vi "Refresh DiffIO Listbox.vi"(4 "_DiffIOState":u8, 5 "AdaptMode":u32, 6 "Results":T1[](array[typedef]) {"Duty Cycle [%]" format="%#_3g"; "Frequency [Hz]" format="%#_3p"}, 7 "DigitalFilter":sgl[](array[numeric]) caption="Filters" format="%#.2p", 8 "Command":T2[](array[typedef]) {"Skip Fire Index" max=7; "Angles"."Duration [s]" format="%#_3p"; "Frequency [Hz]" format="%#_3p"}, 9 "Names":string[](array[string]), 11 "_DiffIO Channels":refnum<vi>) -> ()   [LabVIEW 2016]
uses:
  <vilib>/Powertrain Controls/Device Drivers/DCM/Diff IO/RT/Setup.ctl
  <vilib>/Powertrain Controls/Device Drivers/DCM/Diff IO/FPGA/Mode.ctl
  <vilib>/Powertrain Controls/Device Drivers/DCM/Diff IO/RT/Angle Control.ctl
  <vilib>/Powertrain Controls/Device Drivers/DCM/Diff IO/RT/Results.ctl
  <vilib>/Powertrain Controls/Device Drivers/DCM/Diff IO/RT/DCM - RT - Diff IO.lvlib
  <vilib>/Powertrain Controls/Device Drivers/DCM/Diff IO/FPGA/DCM - FPGA - Diff IO.lvlib
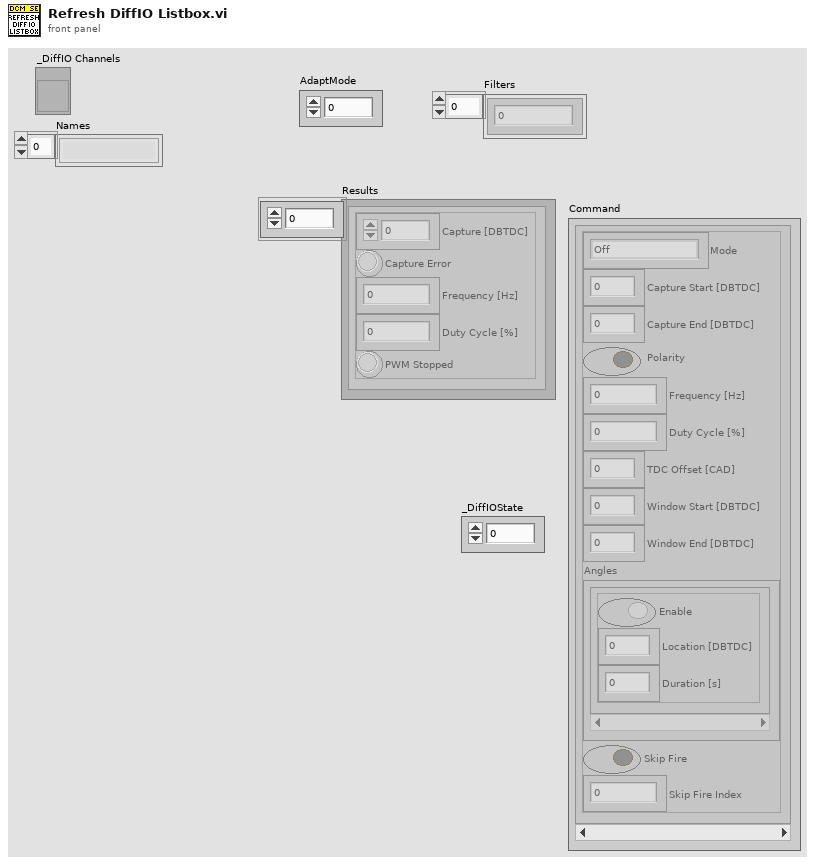
[diagram p1: front panel]
types:
  T1 = typedef "DCM - RT - Diff IO.lvlib/Results.ctl" = cluster{"Capture [DBTDC]":sgl, "Capture Error":bool, "Frequency [Hz]":sgl, "Duty Cycle [%]":sgl, "PWM Stopped":bool}
  T2 = typedef "DCM - RT - Diff IO.lvlib/Setup.ctl" = cluster{"Mode":T3, "Capture Start [DBTDC]":sgl, "Capture End [DBTDC]":sgl, "Polarity":bool, "Frequency [Hz]":sgl, "Duty Cycle [%]":sgl, "TDC Offset [CAD]":sgl, "Window Start [DBTDC]":sgl, "Window End [DBTDC]":sgl, "Angles":T4[], "Skip Fire":bool, "Skip Fire Index":u8}
  T3 = typedef "DCM - FPGA - Diff IO.lvlib/Mode.ctl" = enum8{"Off", "Input", "Pulse Width Modulation", "Engine Position Tracking", "Serial Out 1", "Serial Out 2"}
  T4 = typedef "DCM - RT - Diff IO.lvlib/Angle Control.ctl" = cluster{"Enable":bool, "Location [DBTDC]":sgl, "Duration [s]":sgl}
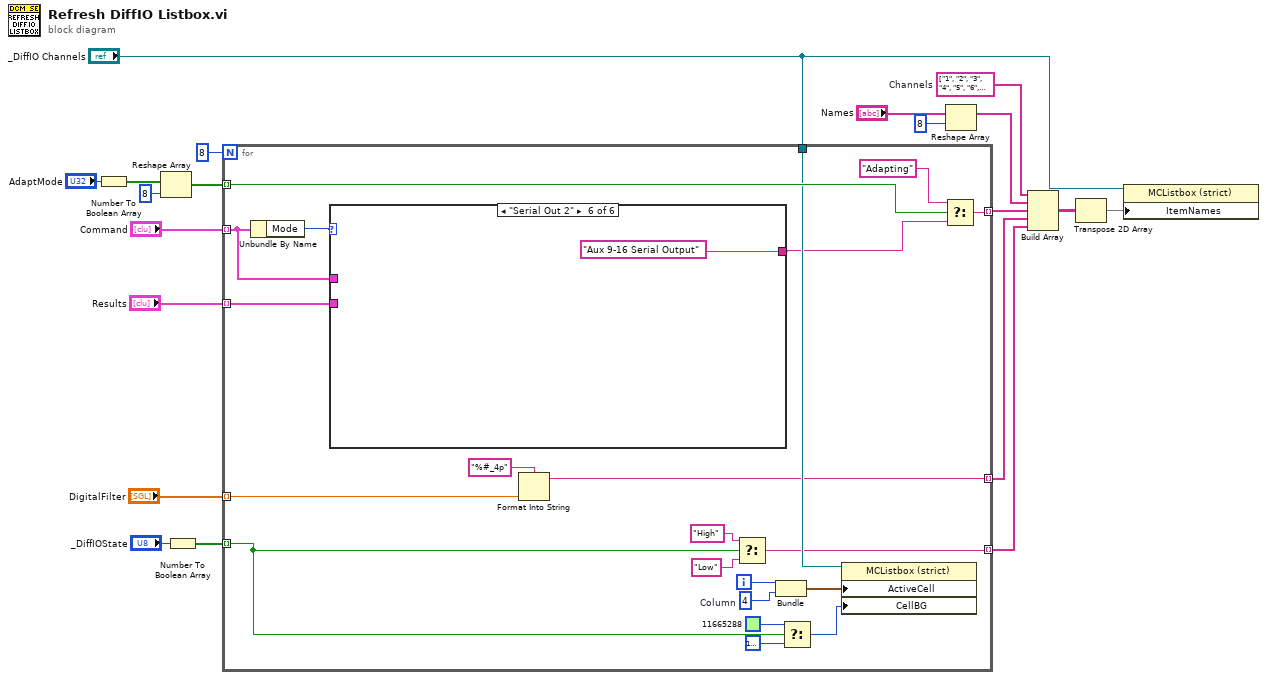
[diagram p0: block diagram]
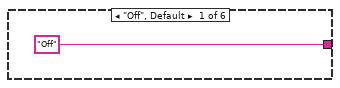
[diagram p2: hidden frame]
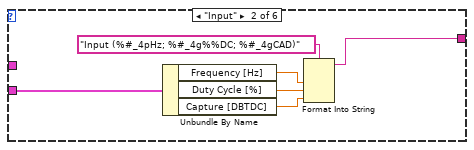
[diagram p3: hidden frame]
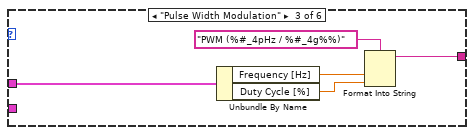
[diagram p4: hidden frame]
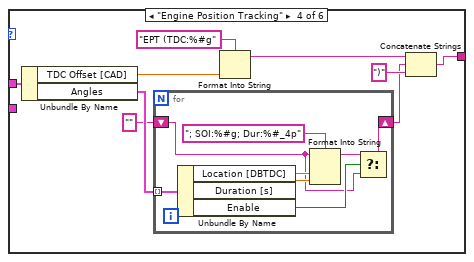
[diagram p5: hidden frame]
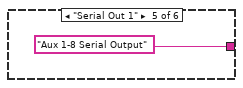
[diagram p6: hidden frame]
diagram:
  w18 = string[] ["1", "2", "3", "4", "5", "6", "7", "8"]  # Channels
  n1 = Number To Boolean Array(number="AdaptMode") -> (Boolean array=w11:bool[])
  n2 = Reshape Array(w11, 8 ("dimension size")) -> (w9:bool[])
  n3 = Number To Boolean Array(number="_DiffIOState") -> (Boolean array=w6:bool[])
  n4 = for {
    N: 8 -> [_]
    tunnel: "Command" -> [w26] mode=indexing
    tunnel: w9 -> [w40] mode=indexing
    tunnel: [w39] -> w8 mode=indexing
    tunnel: "Results" -> [w24] mode=indexing
    tunnel: w6 -> [w29] mode=indexing
    tunnel: [w28] -> w5 mode=indexing
    tunnel: "_DiffIO Channels" -> [w35]
    tunnel: "DigitalFilter" -> [w22] mode=indexing
    tunnel: [w23] -> w1 mode=indexing
    i -> [w37]
    w38 = 4  # Column
    n5 = Unbundle By Name(w26) -> ("Mode"=w27:T3)
    n6 = case shown="\"Serial Out 2\"" w27 {
      tunnel: w26 -> [_ _ w53 w61 _ _]
      tunnel: ["Off" w44 w49 w57 "Aux 1-8 Serial Output" ("format string") "Aux 9-16 Serial Output" ("format string")] -> w25
      tunnel: w24 -> [_ w43 _ _ _ _]
      frame "Off", Default {
      }
      frame "Input" {
        n7 = Unbundle By Name(w43) -> ("Frequency [Hz]"=w46:sgl, "Duty Cycle [%]"=w47:sgl, "Capture [DBTDC]"=w48:sgl)
        n8 = Format Into String(format string="Input (%#_4pHz; %#_4g%%DC; %#_4gCAD)", w46, w47, w48) -> (resulting string=w44:string)  [unwired: 2 in, 1 out]
      }
      frame "Pulse Width Modulation" {
        n9 = Unbundle By Name(w53) -> ("Frequency [Hz]"=w51:sgl, "Duty Cycle [%]"=w50:sgl)
        n10 = Format Into String(format string="PWM (%#_4pHz / %#_4g%%)", w51, w50) -> (resulting string=w49:string)  [unwired: 2 in, 1 out]
      }
      frame "Engine Position Tracking" {
        n11 = Unbundle By Name(w61) -> ("TDC Offset [CAD]"=w60:sgl, "Angles"=w59:T4[])
        n12 = for {
          tunnel: w59 -> [w68] mode=indexing
          shift-right: [w64] -> w55
          shift-left: "" -> [w63]
          n13 = Unbundle By Name(w68) -> ("Location [DBTDC]"=w69:sgl, "Duration [s]"=w67:sgl, "Enable"=w66:bool)
          n14 = Format Into String(format string="; SOI:%#g; Dur:%#_4p", initial string=w63, w69, w67) -> (resulting string=w65:string)  [unwired: 1 in, 1 out]
          n15 = Select(t=w65, s=w66, f=w63) -> (s? t:f=w64:string)
        }
        n16 = Format Into String(format string="EPT (TDC:%#g", w60) -> (resulting string=w58:string)  [unwired: 2 in, 1 out]
        n17 = Concatenate Strings(w58, w55, ")" ("string")) -> (w57:string)
      }
      frame "Serial Out 1" {
      }
      frame "Serial Out 2" {
      }
    }
    n18 = Format Into String(format string="%#_4p", w22) -> (resulting string=w23:string)  [unwired: 2 in, 1 out]
    n19 = Select(t="High" ("format string"), s=w29, f="Low" ("format string")) -> (s? t:f=w28:string)
    n20 = Bundle(w37, "Column"=w38) -> (w36:cluster{i32, "Column":i32})  [unwired: 1 in]
    n21 = Select(t=u32 11665288, s=w29, f=u32 16777226) -> (s? t:f=w32:u32)
    n22 = property on="Property Node" class="MCListbox (strict)"(reference=w35, "ActiveCell"=w36, "CellBG"=w32) -> ()  [unwired: 1 in, 2 out]
    n23 = Select(t="Adapting" ("format string"), s=w40, f=w25) -> (s? t:f=w39:string)
  }
  n24 = Reshape Array("Names", 8 ("dimension size")) -> (w14:string[])
  n25 = Build Array(w18, w14, w8, w1, w5) -> (w20:string[][])
  n26 = Transpose 2D Array(2D array=w20) -> (transposed array=w17:string[][])
  n27 = property on="Property Node" class="MCListbox (strict)"(reference="_DiffIO Channels", "ItemNames"=w17) -> ()  [unwired: 1 in, 2 out]
